vi "2100_Update_Single_Register.vi"(7 "Reg_Address_Data":T1={"Address"=81, "Data"=0} {"Address" format="%.0x"}, 8 "Error In":errorcluster, 11 "Master_Register_Data_Array_In":T2 {"Address" format="%.0x"}) -> (0 "Error Out":errorcluster, 2 "Single_Reg_Address_Data Out":T1={"Address"=81, "Data"=0} {"Address" format="%.0x"}, 3 "Master_Register_Data_Array_Out":T2 {"Address" format="%.0x"})   [LabVIEW 2013]
uses:
  Controls/Master_Reg_Data_Array.ctl
  Controls/Reg_Address_Data.ctl
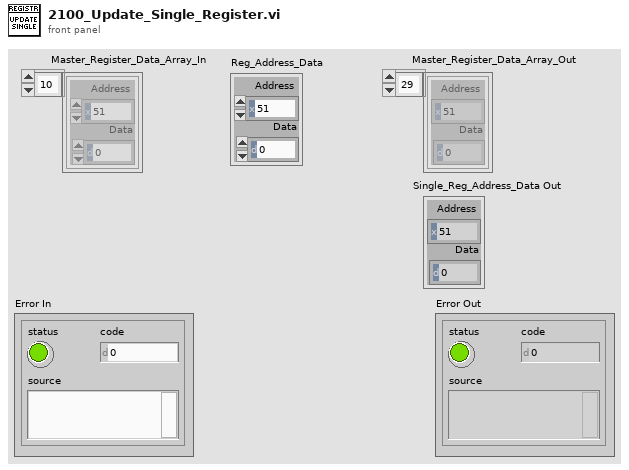
[diagram p1: front panel]
types:
  T1 = typedef "Reg_Address_Data.ctl" = cluster{"Address":u8, "Data":u8}
  T2 = typedef "Master_Reg_Data_Array.ctl" = T1[]
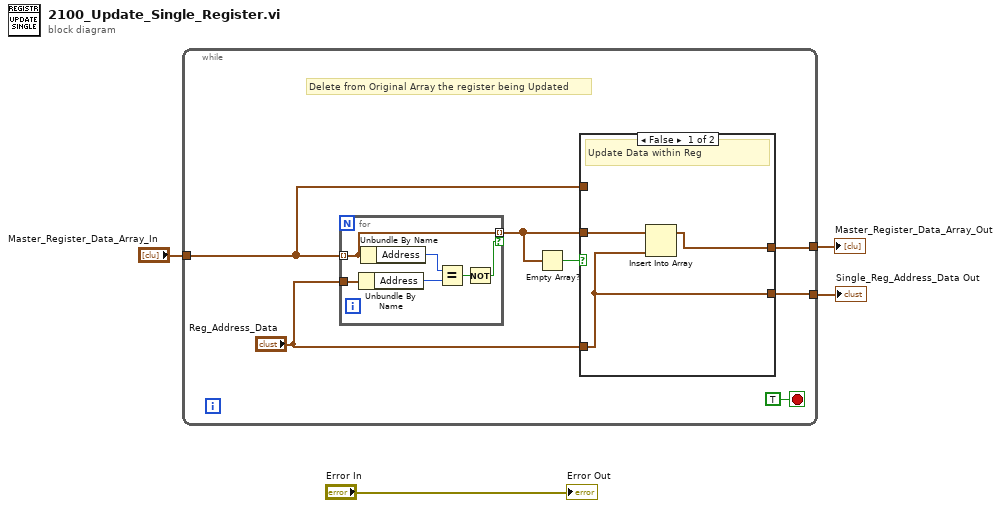
[diagram p0: block diagram]
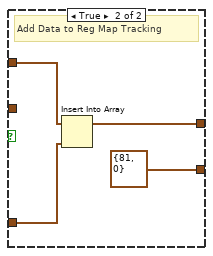
[diagram p2: hidden frame]
diagram:
  n1 = while {
    tunnel: [w10] -> w4
    tunnel: "Master_Register_Data_Array_In" -> [w9]
    tunnel: [w8] -> w1
    stop <- TRUE stop-if-true
    # "Delete from Original Array the register being Updated"
    n2 = for {
      tunnel: w9 -> [w21] mode=indexing
      tunnel: "Reg_Address_Data" -> [w24]
      tunnel: [w21] -> w6 mode=indexing if=w19
      n3 = Unbundle By Name(w24) -> ("Address"=w22:u8)
      n4 = Unbundle By Name(w21) -> ("Address"=w23:u8)
      n5 = Equal?(x=w23, y=w22) -> (x = y?=w20:bool)
      n6 = Not(x=w20) -> (.not. x?=w19:bool)
    }
    n7 = Empty Array?(array=w6) -> (empty?=w5:bool)
    n8 = case shown="False" w5 {
      tunnel: [w14 w17] -> w10
      tunnel: w9 -> [_ w18]
      tunnel: "Reg_Address_Data" -> [w13 w16]
      tunnel: [w13 T1 {"Address"=81, "Data"=0} ("Reg_Address_Data 2")] -> w8
      tunnel: w6 -> [w12 _]
      frame False {
        # "Update Data within Reg"
        n9 = Insert Into Array(array=w12, new element=w13) -> (w14:T1[])  [unwired: 1 in]
      }
      frame True {
        # "Add Data to Reg Map Tracking"
        n10 = Insert Into Array(array=w18, new element=w16) -> (w17:T2)  [unwired: 1 in]
      }
    }
  }
  "Master_Register_Data_Array_Out" <- w4
  "Single_Reg_Address_Data Out" <- w1
  "Error Out" <- "Error In"
